vi "Find Average Center Setup.vi"(4 "Sensor Thickness":dbl, 6 "Assembly Type":string, 8 "Position":i32, 9 "Tray Number":i32, 10 "XYZTheta":dbl[](array[numeric]), 11 "Component":T1) -> (3 "output cluster":T1)   [LabVIEW 2021, in "Component Tray.lvclass"]
uses:
  Component Tray.lvclass
  Find Component.ctl
  Controller/Camera/Machine Vision.ctl
  Controller/Camera/Camera.lvclass
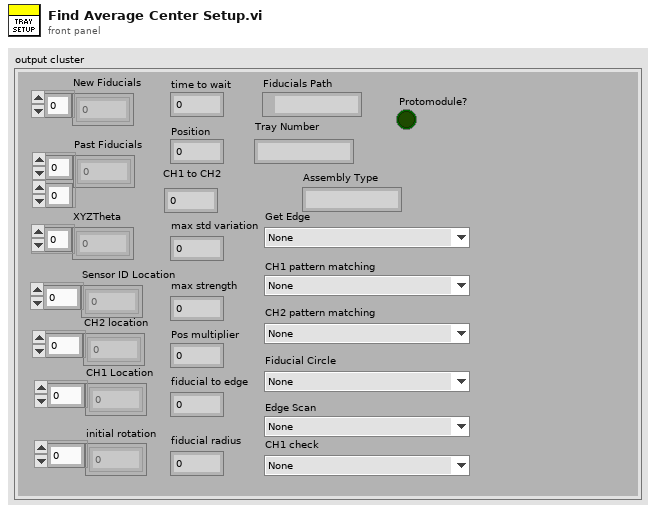
[diagram p1: front panel]
types:
  T1 = typedef "Component Tray.lvclass/Find Component.ctl" = cluster{"New Fiducials":dbl[], "Past Fiducials":dbl[][], "XYZTheta":dbl[], "Fiducials Path":path, "Position":i32, "CH1 Location":dbl[], "Sensor ID Location":dbl[], "initial rotation":dbl[], "CH2 location":dbl[], "max std variation":dbl, "max strength":dbl, "CH2 pattern matching":T2, "Fiducial Circle":T2, "Get Edge":T2, "Pos multiplier":dbl, "time to wait":u32, "fiducial to edge":dbl, "Protomodule?":bool, "Assembly Type":string, "CH1 to CH2":dbl, "Tray Number":string, "fiducial radius":dbl, "4 fiducials?":bool, "CH1 check":T2, "Edge Scan":T2, "CH1 pattern matching":T2, "Sensor Thickness":dbl}
  T2 = typedef "Camera.lvclass/Machine Vision.ctl" = enum16{"None", "Assembly Tray Circle", "Assembly Tray Fiducial", "Partial Hexaboard", "sensor edge init", "HB edge init", "sensor edge pos1", "sensor edge pos2", "HB edge pos1", "HB edge pos2", "Sensor CH1-2", "HB CH1", "HB CH2", "V3 Sensor Circle", "Hexaboard Circle", "sensor CH1 check", "HB CH1 check "}
  T3 = typedef "File Paths.ctl" = cluster{"Glue Pattern Folder":path, "Carrier Tray Folder":path, "Pick Up Tool Fixture Folder":path, "Components Folder":path, "Bellows Tool Offset.txt":path, "Pick Up Tool Offset.txt":path, "Dispense Tip Offset.txt":path, "Log Files":path, "Gantry Assembly Map.txt":path, "Syringe and offset map.txt":path, "Controllers Folder":path, "Local dbase config":path}
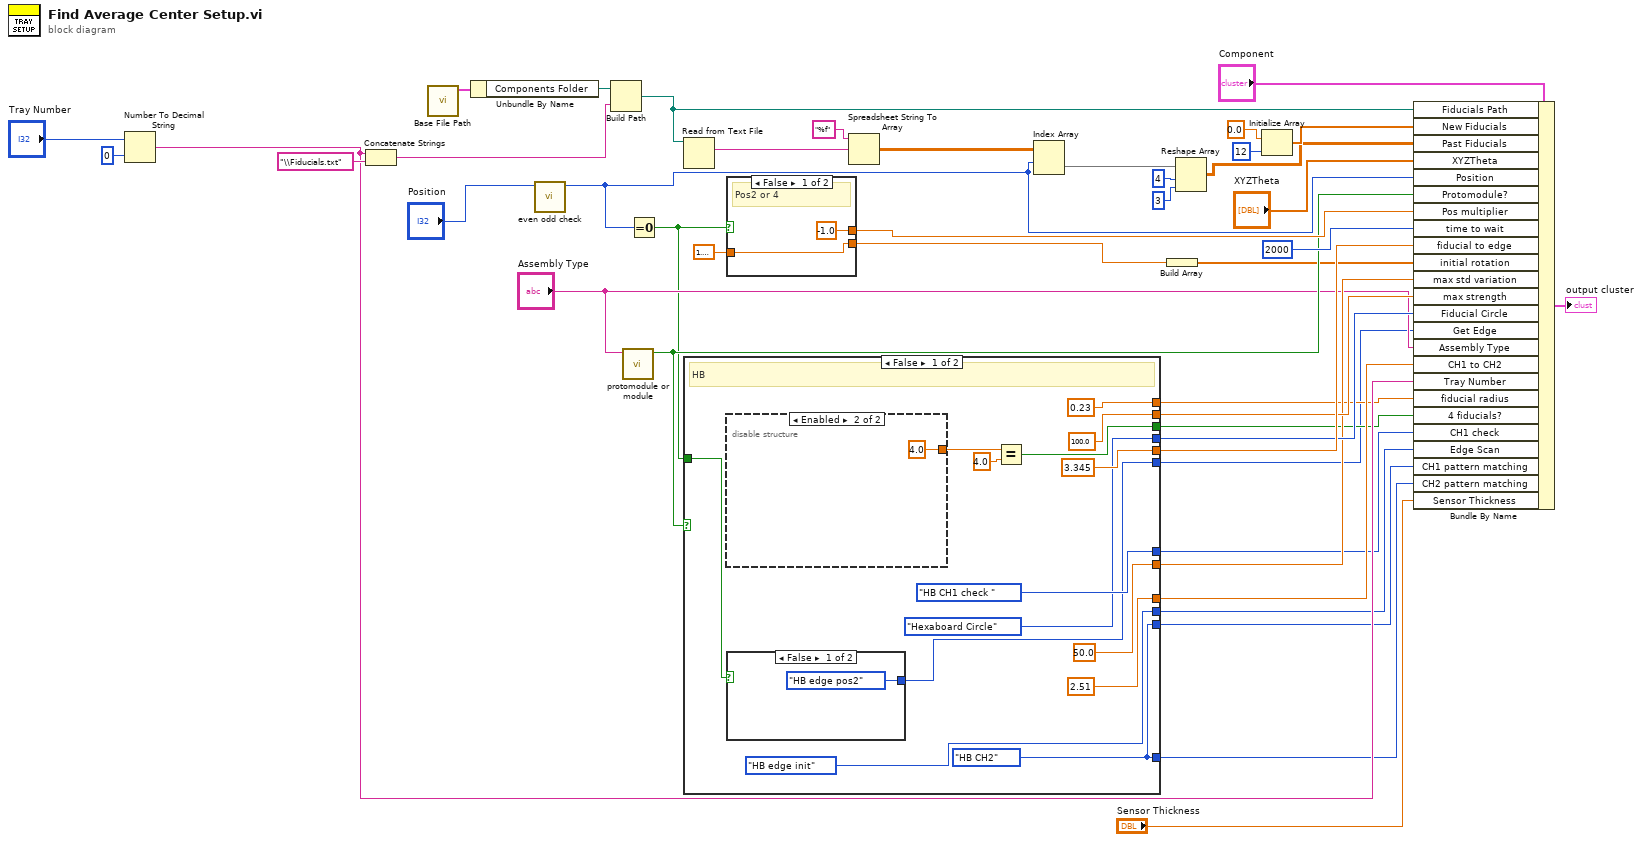
[diagram p0: block diagram]
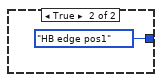
[diagram p2: hidden frame]
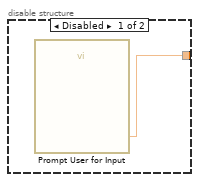
[diagram p3: hidden frame]
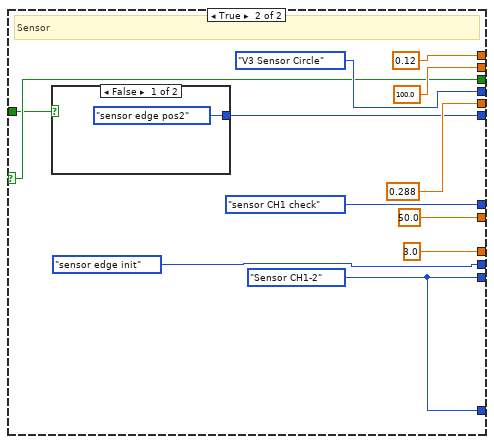
[diagram p4: hidden frame]
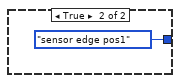
[diagram p5: hidden frame]
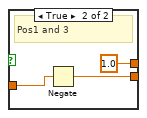
[diagram p6: hidden frame]
diagram:
  n1 = Number To Decimal String(number="Tray Number", width (-)=i16 0) -> (decimal integer string=w10:string)
  n2 = Concatenate Strings "Concatenate Strings"(w10, "\\Fiducials.txt" ("string")) -> (w42:string)
  n3 = call "Base File Path.vi"() -> ("Paths Out"=w38:T3)  [unwired: 11 in]
  n4 = Unbundle By Name(w38) -> ("Components Folder"=w43:path)
  n5 = call "even odd check.vi"("position"="Position") -> ("index"=w22:i32)  [unwired: 10 in]
  n6 = Build Path(base path=w43, name or relative path=w42) -> (appended path=w39:path)
  n7 = call "protomodule or module.vi"("assembly type"="Assembly Type") -> ("protomodule? (T)"=w20:bool)  [unwired: 10 in]
  n8 = Equal To 0?(x=w22) -> (x = 0?=w6:bool)
  n9 = Read from Text File(file (use dialog)=w39) -> (text=w37:string)  [unwired: 3 in, 3 out]
  n10 = case shown="False" w20 {
    selector: w20 -> [_ w69]
    tunnel: [3.345 ("fiducial to edge") 0.288 ("fiducial to edge")] -> w19
    tunnel: [w45 w64] -> w3
    tunnel: [Machine_Vision."Hexaboard Circle" ("Fiducial Circle") Machine_Vision."V3 Sensor Circle" ("Fiducial Circle")] -> w15
    tunnel: [100.0 ("max strength") 100.0 ("max strength")] -> w14
    tunnel: [50.0 ("max std variation") 50.0 ("max std variation")] -> w13
    tunnel: [2.51 ("CH1 to CH2") 3.0 ("CH1 to CH2")] -> w11
    tunnel: [w52 w69] -> w9
    tunnel: [Machine_Vision."HB CH1 check " ("CH1 check") Machine_Vision."sensor CH1 check" ("CH1 check")] -> w8
    tunnel: [0.23 ("fiducial radius") 0.12 ("fiducial radius")] -> w7
    tunnel: w6 -> [w49 w66]
    tunnel: [w48 w65] -> w5
    tunnel: [w45 w64] -> w4
    tunnel: [Machine_Vision."HB edge init" ("Edge Scan") Machine_Vision."sensor edge init" ("Edge Scan")] -> w2
    frame False {
      w45 = Machine_Vision."HB CH2" ("Pattern Matching")
      # "HB"
      n11 = disable-structure shown="Enabled" {
        disable-tunnel: [w61 4.0 ("NumFD")] -> w54
        frame Disabled {
          n12 = call "Prompt User for Input"() -> ("NumFD"=w61:dbl)  [unwired: 17 in, 2 out]
        }
        frame Enabled {
        }
      }
      n13 = case shown="False" w49 {
        tunnel: [Machine_Vision."HB edge pos2" ("Initial Edge") Machine_Vision."HB edge pos1" ("Initial Edge")] -> w48
        frame False {
        }
        frame True {
        }
      }
      n14 = Equal?(x=w54, y=4.0) -> (x = y?=w52:bool)
    }
    frame True {
      w64 = Machine_Vision."Sensor CH1-2" ("Pattern Matching")
      # "Sensor"
      n15 = case shown="False" w66 {
        tunnel: [Machine_Vision."sensor edge pos2" ("Initial Edge") Machine_Vision."sensor edge pos1" ("Initial Edge")] -> w65
        frame False {
        }
        frame True {
        }
      }
    }
  }
  n16 = case shown="False" w6 {
    tunnel: [-1.0 ("Pos multiplier") 1.0 ("Pos multiplier")] -> w23
    tunnel: 1.5707963267948966 -> [w77 w80]
    tunnel: [w77 w79] -> w16
    frame False {
      # "Pos2 or 4"
    }
    frame True {
      # "Pos1 and 3"
      n17 = Negate(x=w80) -> (-x=w79:dbl)
    }
  }
  n18 = Spreadsheet String To Array(format string="%f", spreadsheet string=w37) -> (array=w35:dbl[][])  [unwired: 2 in]
  n19 = Index Array "Index Array"(array=w35, index (row)=w22) -> (element=w34:dbl[])  [unwired: 1 in]
  n20 = Build Array(w16) -> (w18:dbl[])
  n21 = Reshape Array(w34, 4 ("dimension size"), 3 ("dimension size")) -> (w27:dbl[][])
  n22 = Initialize Array(0.0 ("element"), 12 ("dimension size")) -> (w28:dbl[])
  n23 = Bundle By Name "Bundle By Name"(cluster="Component", "Fiducials Path"=w39, "New Fiducials"=w28, "Past Fiducials"=w27, "XYZTheta"="XYZTheta", "Position"=w22, "Protomodule?"=w20, "Pos multiplier"=w23, "time to wait"=u32 2000, "fiducial to edge"=w19, "initial rotation"=w18, "max std variation"=w13, "max strength"=w14, "Fiducial Circle"=w15, "Get Edge"=w5, "Assembly Type"="Assembly Type", "CH1 to CH2"=w11, "Tray Number"=w10, "fiducial radius"=w7, "4 fiducials?"=w9, "CH1 check"=w8, "Edge Scan"=w2, "CH1 pattern matching"=w4, "CH2 pattern matching"=w3, "Sensor Thickness"="Sensor Thickness") -> (→"output cluster":T1)
